vi "Protocol.Convert Frame to NI-XNET CAN Frame.vi"(8 "error in (no error)":errorcluster, 11 "Data to Send":T1 {"Identifier" format="%08x"}) -> (0 "error out":errorcluster, 2 "Source Address":u8, 3 "CAN frame":T2 {"payload" format="%x"; "timestamp" format="%<%.7X\n%x>T"; "type" items=["CAN Data"=0, "CAN Remote"=1, "CAN Bus Error"=2, "CAN 2.0 Data"=8, "CAN FD Data"=16, "CAN FD+BRS Data"=24, "J1939 Data"=192, "Delay"=224, "Log Trigger"=225, "Start Trigger"=226]; "identifier" format="%x"})   [LabVIEW 2023, in "J1939 Addon Engine.lvlib"]
uses:
  J1939 Addon Engine.lvlib
  <vilib>/xnet/xnet.llb/XNET Frame CAN.ctl
  <vilib>/xnet/xnet.llb/XNET Frame Type CAN.ctl
  Support Libraries/J1939 Utilities/Types/CAN Outgoing Message Cluster.ctl
  Support Libraries/J1939 Utilities/J1939 Utilities.lvlib
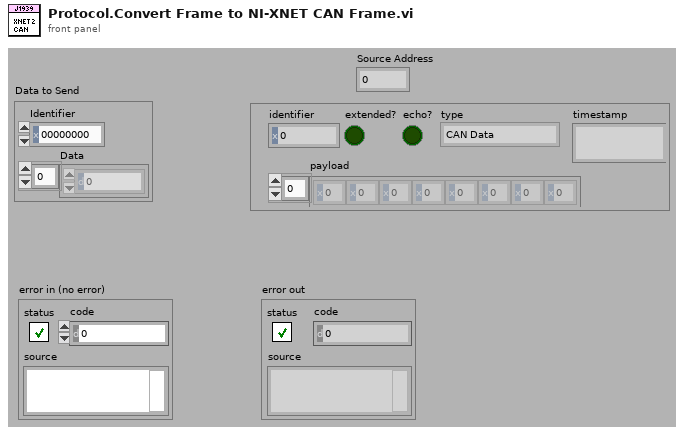
[diagram p1: front panel]
types:
  T1 = typedef "J1939 Utilities.lvlib/CAN Outgoing Message Cluster.ctl" = cluster{"Identifier":u32, "Data":u8[]}
  T2 = typedef "XNET Frame CAN.ctl" = cluster{"timestamp":timestamp, "payload":u8[], "identifier":u32, "type":T3, "extended?":bool, "echo?":bool}
  T3 = typedef "XNET Frame Type CAN.ctl" = u8
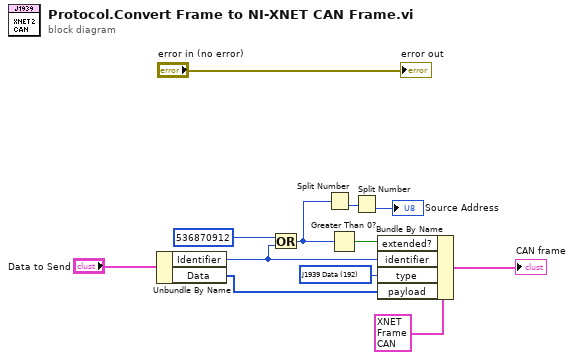
[diagram p0: block diagram]
diagram:
  w2 = T3 192 items=["CAN Data"=0, "CAN Remote"=1, "CAN Bus Error"=2, "CAN 2.0 Data"=8, "CAN FD Data"=16, "CAN FD+BRS Data"=24, "J1939 Data"=192, "Delay"=224, "Log Trigger"=225, "Start Trigger"=226] ("type")
  n1 = Unbundle By Name("Data to Send") -> ("Identifier"=w10:u32, "Data"=w1:u8[])
  n2 = Or(x=u32 536870912, y=w10) -> (x .or. y?=w5:u32)
  n3 = Split Number(x=w5) -> (lo(x)=w6:u16)  [unwired: 1 out]
  n4 = Greater Than 0?(x=w5) -> (x > 0?=w9:bool)
  n5 = Split Number(x=w6) -> (lo(x)=→"Source Address":u8)  [unwired: 1 out]
  n6 = Bundle By Name(cluster=T2 {"timestamp"=timestamp(0 s since 1904-01-01), "payload"=[], "identifier"=0, "type"=0, "extended?"=FALSE, "echo?"=FALSE} ("CAN frame"), "extended?"=w9, "identifier"=w10, "type"=w2, "payload"=w1) -> (→"CAN frame":T2)
  "error out" <- "error in (no error)"
